vi "new RoomWithABomb.vi"(8 "error in (no error)":errorcluster, 10 "roomNumber":i32) -> (0 "error out":errorcluster, 3 "RoomWithABomb* out":T1)   [LabVIEW 2016, in "RoomWithABomb.lvclass"]
uses:
  RoomWithABomb.lvclass
  RoomWithABomb Reference.ctl
  C:/github/LVOOP-creational-patterns/Maze-Classes/src/Base/Room/Room.lvclass
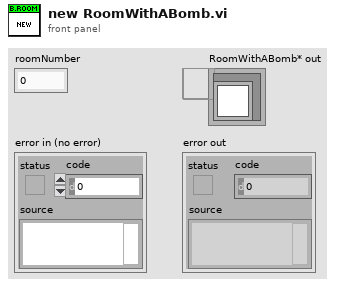
[diagram p1: front panel]
types:
  T1 = typedef "RoomWithABomb.lvclass/RoomWithABomb Reference.ctl" = refnum<data-value>
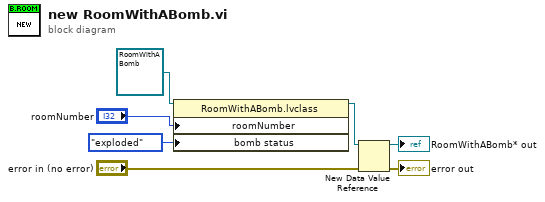
[diagram p0: block diagram]
diagram:
  n1 = property class="RoomWithABomb.lvclass"(reference=refnum<class "RoomWithABomb.lvclass"> refnum ("RoomWithABomb in"), "roomNumber"="roomNumber", "bomb status"=enum16{"none", "exploded", "unexploded"}."exploded") -> (reference out=w4:refnum<class "RoomWithABomb.lvclass">)  [unwired: 1 in, 1 out]
  n2 = New Data Value Reference(data value=w4, error in="error in (no error)") -> (data value reference=→"RoomWithABomb* out":refnum<data-value>, error out=→"error out":errorcluster)
